vi "sub_main_appcomm.vi"(8 "error in":errorcluster) -> (0 "error out":errorcluster)   [LabVIEW 2019]
panel:
  out "receive":string
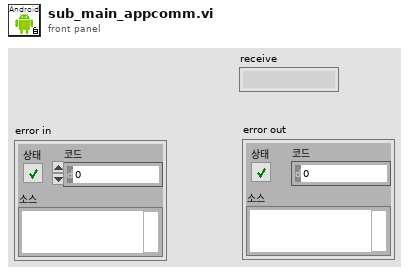
[diagram p1: front panel]
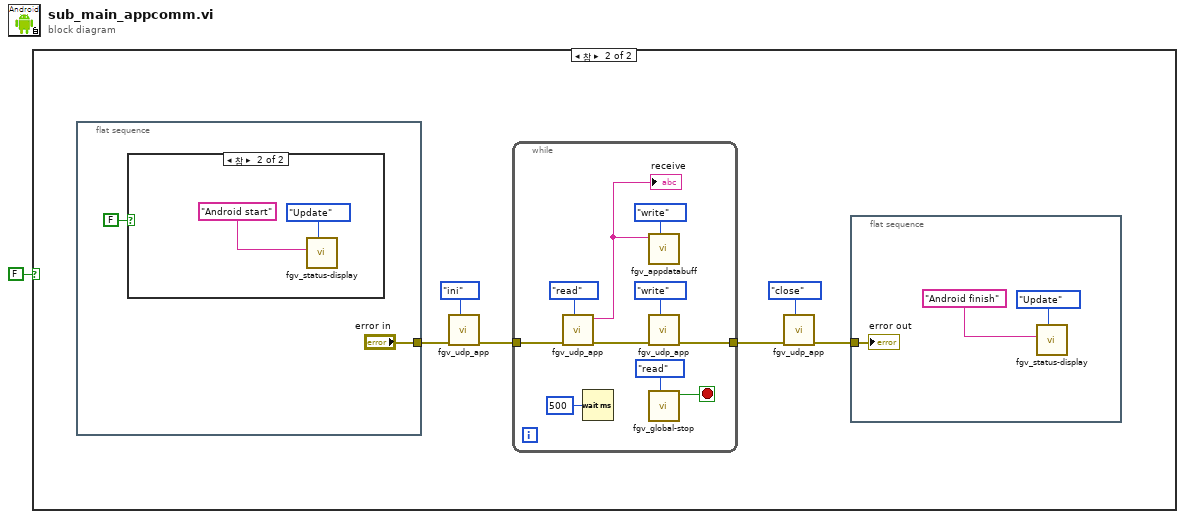
[diagram p0: block diagram]
diagram:
  n1 = case shown="참" FALSE {
    frame False {
    }
    frame True {
      n2 = flat-sequence {
        tunnel: ["error in"] -> w6
        frame #0 {
          n3 = case shown="참" FALSE {
            frame False {
            }
            frame True {
              n4 = call "fgv_status-display.vi"("Mode"=enum16{"Initial", "Update", "Clear"}."Update", "title"="Android start" ("String in 1")) -> ()  [unwired: 9 in, 1 out]
            }
          }
        }
      }
      n5 = call "fgv_udp_app.vi"("cmd"=enum16{"ini", "write", "read", "close"}."ini", "error in"=w6) -> ("error out"=w4:errorcluster)  [unwired: 8 in, 1 out]
      n6 = while {
        tunnel: w4 -> [w22]
        tunnel: [w20] -> w5
        stop <- w16 stop-if-true
        n7 = call "fgv_udp_app.vi"("cmd"=enum16{"ini", "write", "read", "close"}."read", "error in"=w22) -> ("error out"=w21:errorcluster, "receive"=w18:string)  [unwired: 8 in]
        "receive" <- w18
        n8 = Wait (ms)(milliseconds to wait=u32 500 ("대기 시간 (ms)")) -> ()  [unwired: 1 out]
        n9 = call "fgv_appdatabuff.vi"("cmd"=enum16{"read", "write"}."write", "receive str in"=w18) -> ()  [unwired: 9 in, 1 out]
        n10 = call "fgv_udp_app.vi"("cmd"=enum16{"ini", "write", "read", "close"}."write", "error in"=w21) -> ("error out"=w20:errorcluster)  [unwired: 8 in, 1 out]
        n11 = call "fgv_global-stop.vi"("cmd"=enum16{"init", "stop", "read"}."read") -> ("val_out"=w16:bool)  [unwired: 10 in]
      }
      n12 = call "fgv_udp_app.vi"("cmd"=enum16{"ini", "write", "read", "close"}."close", "error in"=w5) -> ("error out"=w7:errorcluster)  [unwired: 8 in, 1 out]
      n13 = flat-sequence {
        tunnel: w7 -> [w10]
        frame #0 {
          n14 = call "fgv_status-display.vi"("Mode"=enum16{"Initial", "Update", "Clear"}."Update", "title"="Android finish" ("String in 1")) -> ()  [unwired: 9 in, 1 out]
          "error out" <- w10
        }
      }
    }
  }
